vi "Destroy DSF Configuration Session v2.vi"(8 "error in (no error)":errorcluster, 11 "config data ref":T1) -> (0 "error out":errorcluster)   [LabVIEW 2017, in "DSF Configuration.lvlib" / "Configuration Session.lvclass"]
uses:
  Configuration Session.lvclass
  Config Data Ref.ctl
  DSF Configuration API/Private/Controls/Session/DSF Config Data.ctl
  DSF Configuration API/Private/Controls/DSF File Format/Internal.DSF Configuration.ctl
  DSF Configuration API/Public/Controls/DSF Version Info.ctl
  DSF Configuration API/Private/Controls/DSF File Format/Internal.DSF Plugin with ID.ctl
  DSF Configuration API/Private/Controls/DSF File Format/Internal.DSF Plugin Info.ctl
  DSF Configuration API/Public/Controls/DSF Timing Info.ctl
  DSF Configuration API/Private/Controls/DSF File Format/Internal.DSF Group with ID.ctl
  DSF Configuration API/Private/Controls/DSF File Format/Internal.DSF Group Info.ctl
  DSF Configuration API/Private/Controls/DSF File Format/Internal.DSF Transfer with ID.ctl
  DSF Configuration API/Private/Controls/DSF File Format/Internal.DSF Transfer Info.ctl
  DSF Configuration API/Private/Controls/DSF File Format/Internal.DSF Channel with ID.ctl
  DSF Configuration API/Private/Controls/DSF File Format/Internal.DSF Channel Info.ctl
  DSF Configuration API/Private/Controls/DSF File Format/Internal.DSF Settings with ID.ctl
  DSF Configuration API/Private/Controls/DSF File Format/Internal.DSF Settings Info.ctl
  DSF Configuration.lvlib
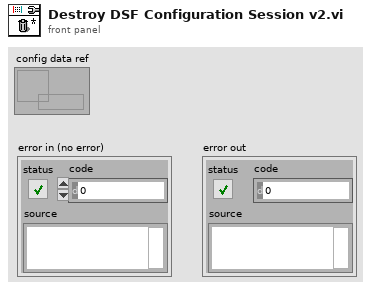
[diagram p1: front panel]
types:
  T1 = typedef "DSF Configuration.lvlib/Configuration Session.lvclass/Config Data Ref.ctl" = refnum<data-value>
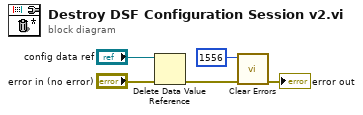
[diagram p0: block diagram]
diagram:
  n1 = Delete Data Value Reference(data value reference="config data ref", error in="error in (no error)") -> (error out=w5:errorcluster)  [unwired: 1 out]
  n2 = call <vilib>:"Clear Errors.vi"("error in (no error)"=w5, "specific error code to clear (0: all)"=1556) -> ("error out"=→"error out":errorcluster)  [unwired: 4 in, 1 out]
